vi "CreateCommand.vi"(8 "Default Data":variant, 9 "Acceptable Robot States":string[](array[string]), 10 "Interruptable":bool, 11 "Name":string) -> (3 "Command":T1)   [LabVIEW 2017]
uses:
  <userlib>/836-Library/Robot/Command/Support/CommandType.ctl
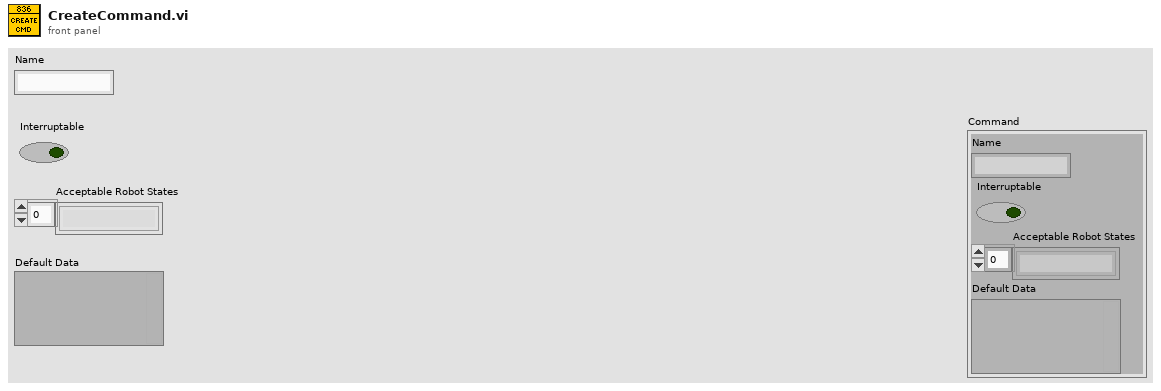
[diagram p1: front panel]
types:
  T1 = typedef "CommandType.ctl" = cluster{"Name":string, "Interruptable":bool, "Acceptable Robot States":string[], "Default Data":variant}
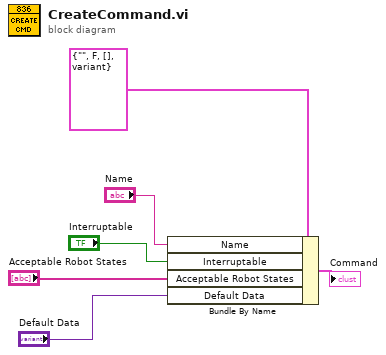
[diagram p0: block diagram]
diagram:
  n1 = Bundle By Name(cluster=T1 {"Name"="", "Interruptable"=FALSE, "Acceptable Robot States"=[], "Default Data"=variant} ("Command"), "Name"="Name", "Interruptable"="Interruptable", "Acceptable Robot States"="Acceptable Robot States", "Default Data"="Default Data") -> (→"Command":T1)
